vi "Prepare Pattern.vi"(11 "Pattern":string) -> (3 "Prepared Pattern":string)   [LabVIEW 2017]
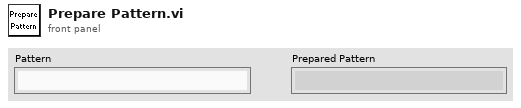
[diagram p1: front panel]
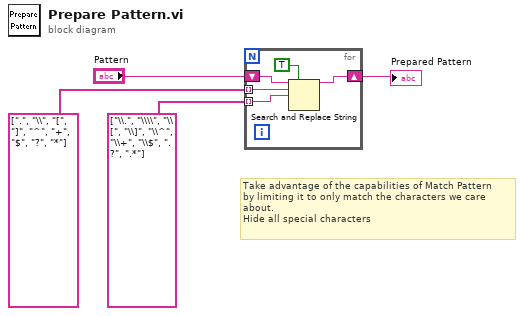
[diagram p0: block diagram]
diagram:
  # "Take advantage of the capabilities of Match Pattern\nby limiting it to only match the characters we care\nabout.\nHide all special characters"
  n1 = for {
    shift-right: [w8] -> w1
    shift-left: "Pattern" -> [w9]
    tunnel: string[] [".", "\\", "[", "]", "^", "+", "$", "?", "*"] -> [w7] mode=indexing
    tunnel: string[] ["\\.", "\\\\", "\\[", "\\]", "\\^", "\\+", "\\$", ".?", ".*"] -> [w6] mode=indexing
    n2 = Search and Replace String(replace all?=TRUE, input string=w9, search string=w7, replace string=w6) -> (result string=w8:string)  [unwired: 4 in, 3 out]
  }
  "Prepared Pattern" <- w1
